vi "Verify Font Name, Encoding and Size.vi"(10 "Font IN":T1={"Name"="", "Size"=-1.0, "Color"=0, "Style"={"Bold"=FALSE, "Italic"=FALSE, "Underline"=FALSE, "Strikeout"=FALSE}, "Type"={"Type&direction"=enum."Select", "Embedded"=FALSE, "Encoding"=""}}, 11 "Default Font cluster":T1={"Name"="STSONG", "Size"=12.0, "Color"=0, "Style"={"Bold"=FALSE, "Italic"=FALSE, "Underline"=FALSE, "Strikeout"=FALSE}, "Type"={"Type&direction"=enum."Select", "Embedded"=FALSE, "Encoding"=""}}) -> (2 "Font OUT":T1={"Name"="Helvetica", "Size"=12.0, "Color"=0, "Style"={"Bold"=FALSE, "Italic"=FALSE, "Underline"=FALSE, "Strikeout"=FALSE}, "Type"={"Type&direction"=enum."Select", "Embedded"=FALSE, "Encoding"=""}}, 3 "Font = default font":bool)   [LabVIEW 2020, in "Exaprom PDF.lvlib" / "Font Class.lvclass"]
doc: "Version 1.1\nDeveloped by Jean-Marc Simard\nCopyright © 2013, Exaprom Inc.\nAll rights reserved.\nLicense: BSD"
uses:
  <userlib>/labview-PDF-writer-master/LV Class/Fonts Class/Font Class.lvclass
  <userlib>/labview-PDF-writer-master/Controls/Font Controls/Font complete cluster.ctl
  <userlib>/labview-PDF-writer-master/Controls/Font Controls/Font size.ctl
  <userlib>/labview-PDF-writer-master/Controls/Font Controls/Font color.ctl
  <userlib>/labview-PDF-writer-master/Controls/Font Controls/Type and encoding.ctl
  <userlib>/labview-PDF-writer-master/Controls/Text Controls/Unicode/Type and run direction.ctl
  <userlib>/labview-PDF-writer-master/Exaprom PDF.lvlib
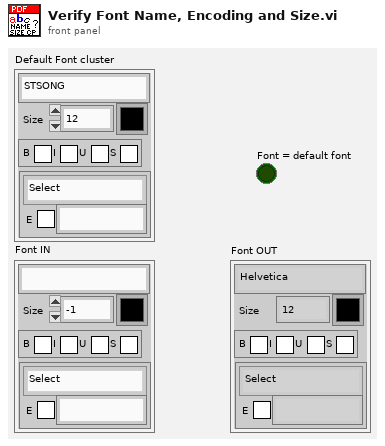
[diagram p1: front panel]
types:
  T1 = typedef "Exaprom PDF.lvlib/Font complete cluster.ctl" = cluster{"Name":string, "Size":T2, "Color":T3, "Style":cluster{"Bold":bool, "Italic":bool, "Underline":bool, "Strikeout":bool}, "Type":T4}
  T2 = typedef "Exaprom PDF.lvlib/Font size.ctl" = sgl
  T3 = typedef "Exaprom PDF.lvlib/Font color.ctl" = u32
  T4 = typedef "Exaprom PDF.lvlib/Type and encoding.ctl" = cluster{"Type&direction":T5, "Embedded":bool, "Encoding":string}
  T5 = typedef "Exaprom PDF.lvlib/Type and run direction.ctl" = enum16{"Select", "ASCII", "UTF-16", "UTF-16 (default)", "UTF-16 (LTR)", "UTF-16 (RTL)"}
  T6 = cluster{"Name":string, "Size":T2, "Color":T3, "Style":cluster{"Bold":bool, "Italic":bool, "Underline":bool, "Strikeout":bool}, "Encoding":string}
  T7 = cluster{"Bold":bool, "Italic":bool, "Underline":bool, "Strikeout":bool}
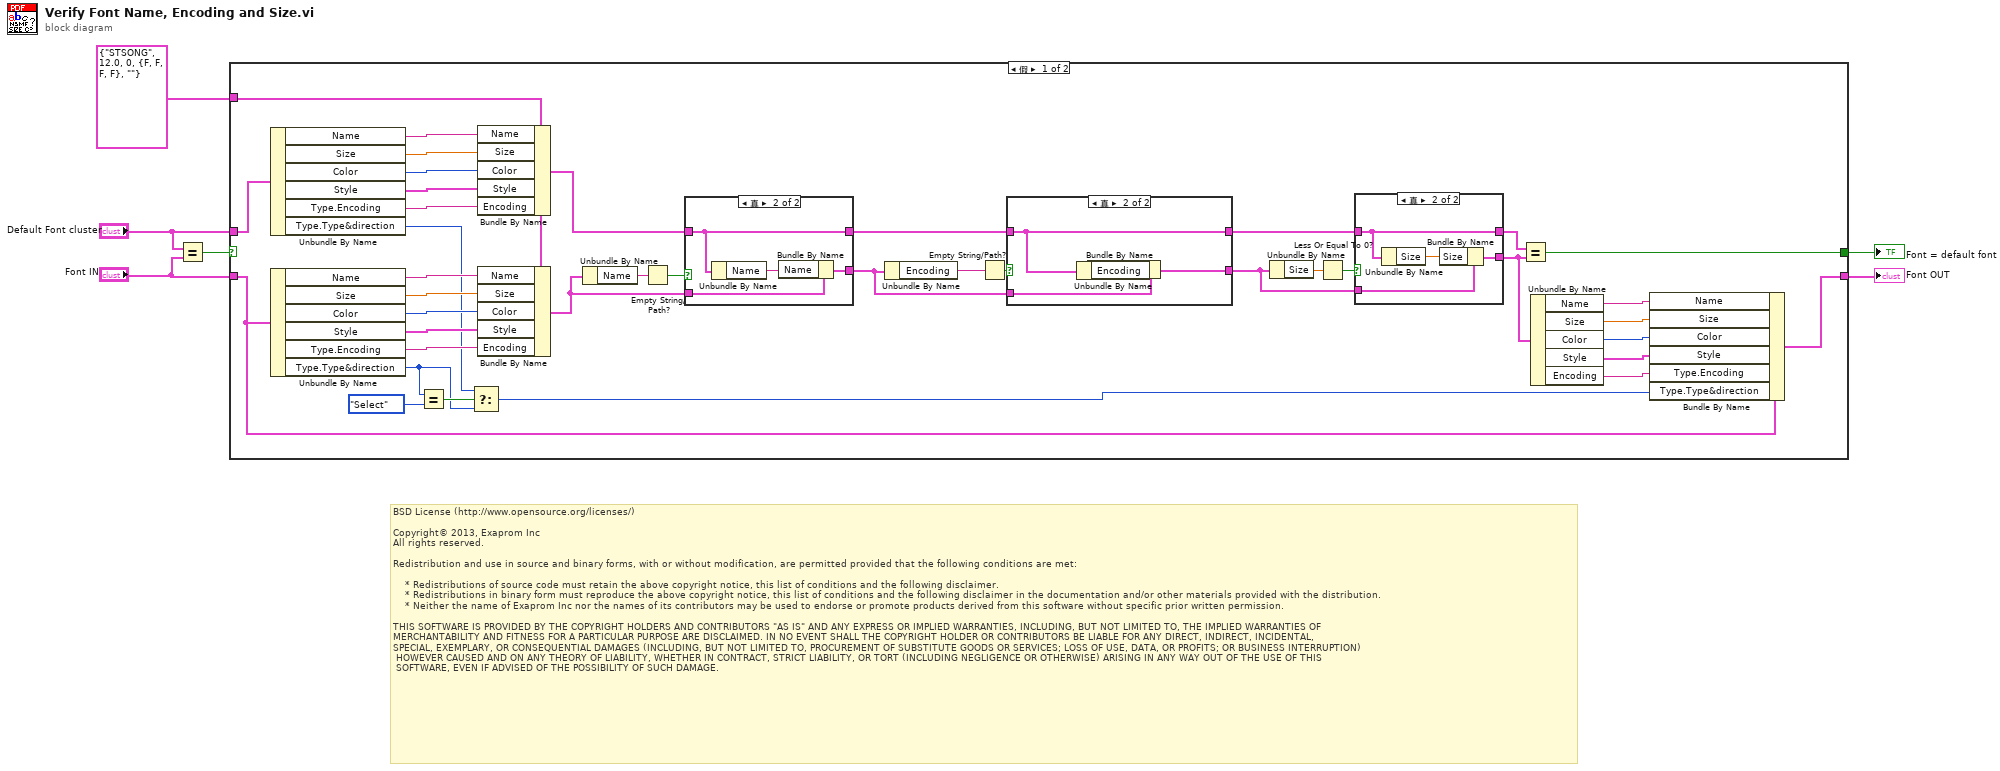
[diagram p0: block diagram]
diagram:
  # "BSD License (http://www.opensource.org/licenses/)\n\nCopyright© 2013, Exaprom Inc\nAll rights reserved.\n\nRedistribution and use in source and binary forms, with or without modification, are permitted provided that the following conditions are met:\n\n    * Redistributions of source code must retain the above copyright notice, this list of conditions and the following disclaimer.\n    * Redistributions in binary form must reproduce the above copyright notice, this list of conditions and the following disclaimer in the documentation and/or other materials provided with the distribution.\n    * Neither the name of Exaprom Inc nor the names of its contributors may be used to endorse or promote products derived from this software without specific prior written permission.\n\nTHIS SOFTWARE IS PROVIDED BY THE COPYRIGHT HOLDERS AND CONTRIBUTORS \"AS IS\" AND ANY EXPRESS OR IMPLIED WARRANTIES, INCLUDING, BUT NOT LIMITED TO, THE IMPLIED WARRANTIES OF \nMERCHANTABILITY AND FITNESS FOR A PARTICULAR PURPOSE ARE DISCLAIMED. IN NO EVENT SHALL THE COPYRIGHT HOLDER OR CONTRIBUTORS BE LIABLE FOR ANY DIRECT, INDIRECT, INCIDENTAL,\nSPECIAL, EXEMPLARY, OR CONSEQUENTIAL DAMAGES (INCLUDING, BUT NOT LIMITED TO, PROCUREMENT OF SUBSTITUTE GOODS OR SERVICES; LOSS OF USE, DATA, OR PROFITS; OR BUSINESS INTERRUPTION)\n HOWEVER CAUSED AND ON ANY THEORY OF LIABILITY, WHETHER IN CONTRACT, STRICT LIABILITY, OR TORT (INCLUDING NEGLIGENCE OR OTHERWISE) ARISING IN ANY WAY OUT OF THE USE OF THIS\n SOFTWARE, EVEN IF ADVISED OF THE POSSIBILITY OF SUCH DAMAGE."
  n1 = Equal?(x="Default Font cluster", y="Font IN") -> (x = y?=w6:bool)
  n2 = case shown="假" w6 {
    selector: w6 -> [_ w65]
    tunnel: "Default Font cluster" -> [w28 _]
    tunnel: "Font IN" -> [w14 w64]
    tunnel: [w41 w65] -> w3
    tunnel: [w7 w64] -> w2
    tunnel: T6 {"Name"="STSONG", "Size"=12.0, "Color"=0, "Style"={"Bold"=FALSE, "Italic"=FALSE, "Underline"=FALSE, "Strikeout"=FALSE}, "Encoding"=""} ("Default Font cluster") -> [w20 _]
    frame False {
      n3 = Unbundle By Name(w28) -> ("Name"=w33:string, "Size"=w32:T2, "Color"=w31:T3, "Style"=w30:T7, "Type.Encoding"=w29:string, "Type.Type&direction"=w17:T5)
      n4 = Unbundle By Name(w14) -> ("Name"=w22:string, "Size"=w23:T2, "Color"=w24:T3, "Style"=w25:T7, "Type.Encoding"=w26:string, "Type.Type&direction"=w16:T5)
      n5 = Equal?(x=w16, y=Type_and_run_direction."Select") -> (x = y?=w18:bool)
      n6 = Select(t=w17, s=w18, f=w16) -> (s? t:f=w8:T5)
      n7 = Bundle By Name(cluster=w20, "Name"=w33, "Size"=w32, "Color"=w31, "Style"=w30, "Encoding"=w29) -> (w27:T6)
      n8 = Bundle By Name(cluster=w20, "Name"=w22, "Size"=w23, "Color"=w24, "Style"=w25, "Encoding"=w26) -> (w21:T6)
      n9 = Unbundle By Name(w21) -> ("Name"=w45:string)
      n10 = Empty String/Path?(string/path=w45) -> (empty?=w44:bool)
      n11 = case shown="真" w44 {
        tunnel: w21 -> [w59 w62]
        tunnel: w27 -> [w58 w60]
        tunnel: [w59 w61] -> w37
        tunnel: [w58 w60] -> w38
        frame False {
        }
        frame True {
          n12 = Unbundle By Name(w60) -> ("Name"=w63:string)
          n13 = Bundle By Name(cluster=w62, "Name"=w63) -> (w61:T6)
        }
      }
      n14 = Unbundle By Name(w37) -> ("Encoding"=w39:string)
      n15 = Empty String/Path?(string/path=w39) -> (empty?=w40:bool)
      n16 = case shown="真" w40 {
        tunnel: w37 -> [w47 w50]
        tunnel: w38 -> [w46 w48]
        tunnel: [w47 w49] -> w36
        tunnel: [w46 w48] -> w35
        frame False {
        }
        frame True {
          n17 = Unbundle By Name(w48) -> ("Encoding"=w51:string)
          n18 = Bundle By Name(cluster=w50, "Encoding"=w51) -> (w49:T6)
        }
      }
      n19 = Unbundle By Name(w36) -> ("Size"=w43:T2)
      n20 = Less Or Equal To 0?(x=w43) -> (x <= 0?=w42:bool)
      n21 = case shown="真" w42 {
        tunnel: w36 -> [w53 w57]
        tunnel: w35 -> [w52 w54]
        tunnel: [w53 w55] -> w15
        tunnel: [w52 w54] -> w34
        frame False {
        }
        frame True {
          n22 = Unbundle By Name(w54) -> ("Size"=w56:T2)
          n23 = Bundle By Name(cluster=w57, "Size"=w56) -> (w55:T6)
        }
      }
      n24 = Equal?(x=w34, y=w15) -> (x = y?=w41:bool)
      n25 = Unbundle By Name(w15) -> ("Name"=w13:string, "Size"=w12:T2, "Color"=w11:T3, "Style"=w10:T7, "Encoding"=w9:string)
      n26 = Bundle By Name(cluster=w14, "Name"=w13, "Size"=w12, "Color"=w11, "Style"=w10, "Type.Encoding"=w9, "Type.Type&direction"=w8) -> (w7:T1)
    }
    frame True {
    }
  }
  "Font = default font" <- w3
  "Font OUT" <- w2
